vi "Push_Data_Front_Pannel.vi"(9 "清除原有数据":bool, 10 "错误输入（无错误）":errorcluster, 11 "数组":string[][](array[string])) -> ()   [LabVIEW 2016]
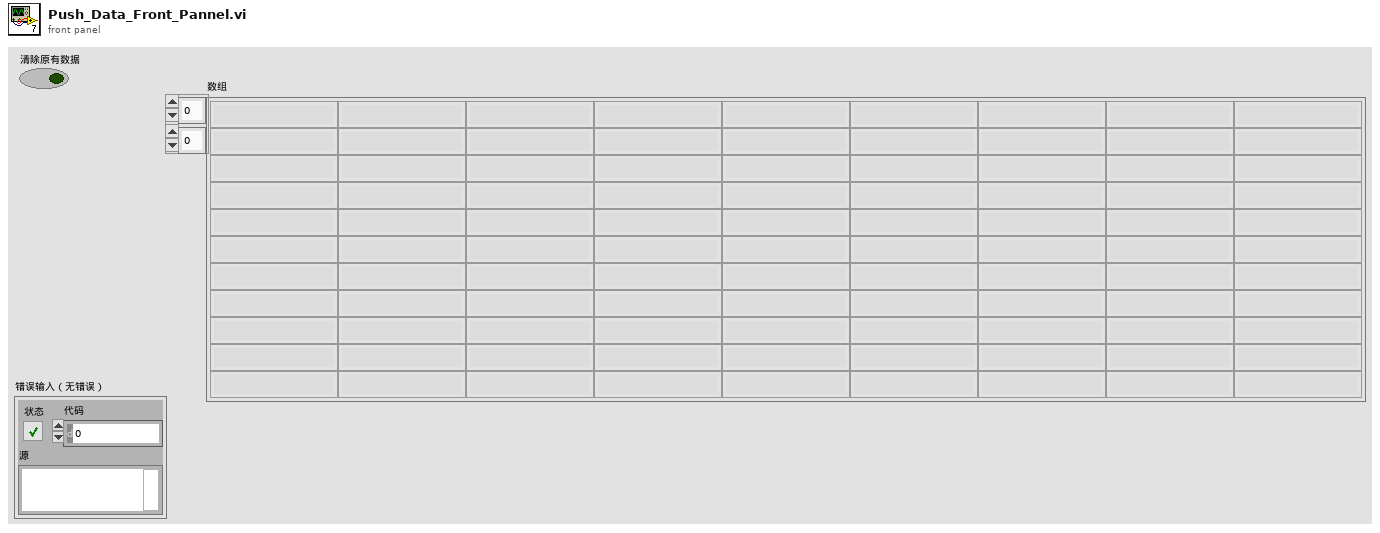
[diagram p1: front panel]
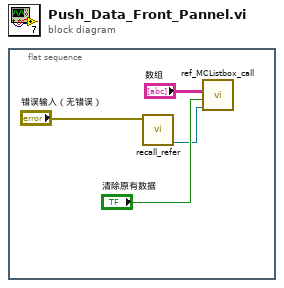
[diagram p0: block diagram]
diagram:
  n1 = flat-sequence {
    frame #0 {
      n2 = call "recall_refer.vi"("错误输入（无错误）"="错误输入（无错误）") -> ("引用输出"=w1:refnum<vi>)  [unwired: 8 in, 2 out]
      n3 = call "ref_MCListbox_call.vi"("VI引用输入"=w1, "清除原有数据"="清除原有数据", "数组"="数组") -> ()  [unwired: 9 in]
    }
  }
